vi "SMU Output Connection Control .vi"(7 "output connected?":bool=TRUE caption="output enabled", 8 "error in (no error)":errorcluster, 10 "Pins":string[](array[string])=["VIO", "VP", "HV"], 11 "Semiconductor Module Context":T1) -> (0 "error Out":errorcluster)   [LabVIEW 2013]
uses:
  <vilib>/NI_TestStand_SemiconductorModule/NI_TestStand_Semiconductor_Module.lvlibp/PinMap/General/SemiconductorModuleContext.ctl
  <vilib>/NI_TestStand_SemiconductorModule/NI_TestStand_Semiconductor_Module.lvlibp/PinMap/DC Power/PinsToNIDCPowerSessions.vi
  <vilib>/NI_TestStand_SemiconductorModule/NI_TestStand_Semiconductor_Module.lvlibp
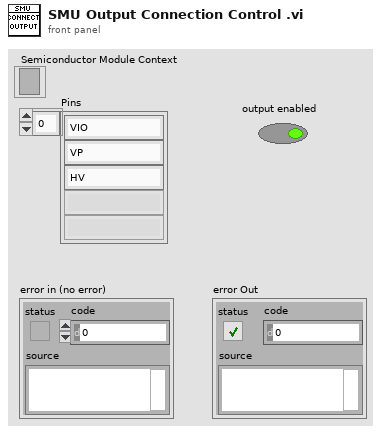
[diagram p1: front panel]
types:
  T1 = typedef "NI_TestStand_Semiconductor_Module.lvlibp/SemiconductorModuleContext.ctl" = refnum<k7>
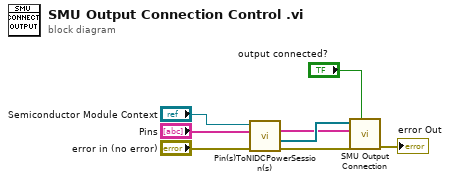
[diagram p0: block diagram]
diagram:
  n1 = call-poly <vilib>:"Pin(s)ToNIDCPowerSession(s).vi"("error in (no error)"="error in (no error)", "Pins"="Pins", "Semiconductor Module Context"="Semiconductor Module Context") -> ("error out"=w5:errorcluster, "Instrument Sessions"=w2:refnum<k15>[], "Channel Lists"=w1:string[])  [unwired: 4 in, 2 out]
  n2 = call "SMU Output Connection.vi"("output enabled"="output connected?", "error in (no error)"=w5, "Channel Lists"=w1, "Instrument Sessions In"=w2) -> ("error Out"=→"error Out":errorcluster)  [unwired: 6 in, 1 out]
